vi "autoMotionProfileGenerate.vi"(11 "InputCommand":string[](array[string])) -> (2 "Acceleration steps (ft/s^2)":dbl[](array[numeric]), 3 "Speed steps (ft/s)":dbl[](array[numeric]))   [LabVIEW 2013]
panel:
  in  "autoTimeDelay":dbl
  out "Array of Computational Values":dbl[][](array[numeric])
  out "Array 2":dbl[](array[numeric])
  out "# of F2 Terms":dbl
  out "Total # of Steps":dbl
  out "# of F1 Terms":dbl
  out "N (# of steps)":dbl
  in  "T2 (s)":dbl
  in  "T1 (s)":dbl
  in  "Distance (ft)":dbl
  in  "Vprog (ft/s)":dbl
  # "Requires array slots 8, 9, 10, 11\nto be Vprog, distance, T1, T2"
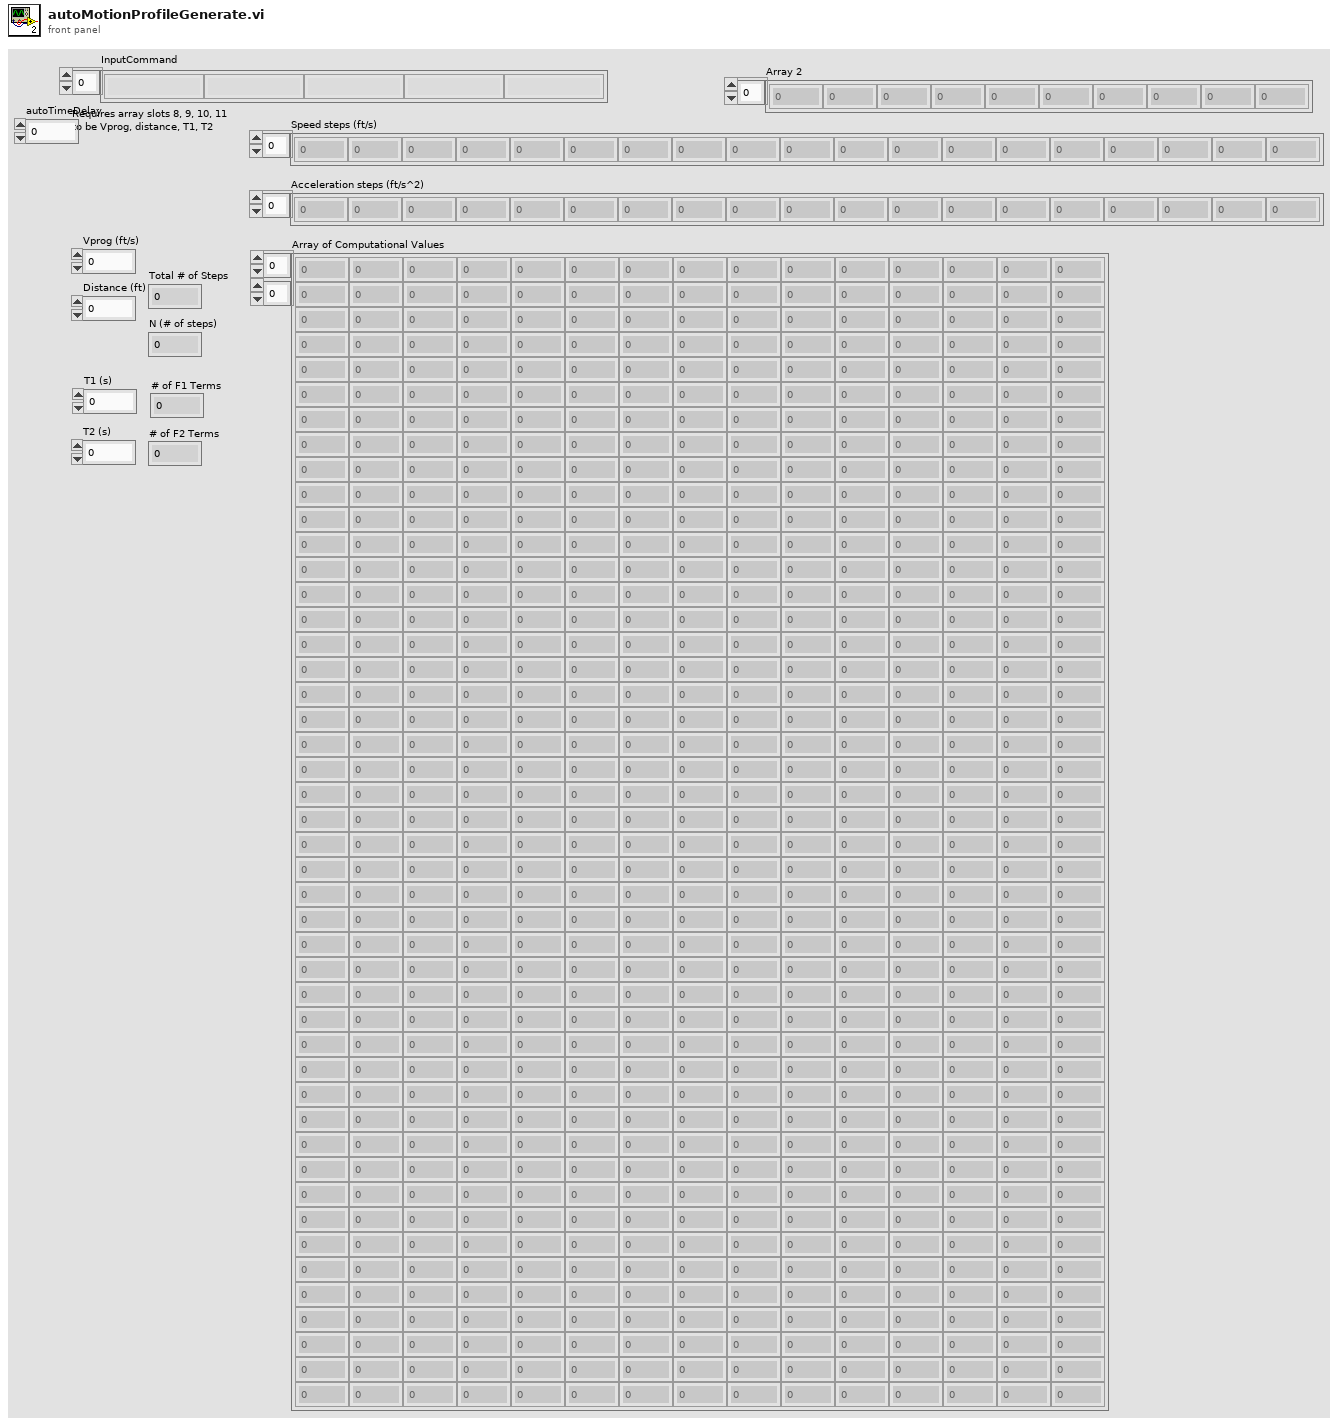
[diagram p1: front panel]
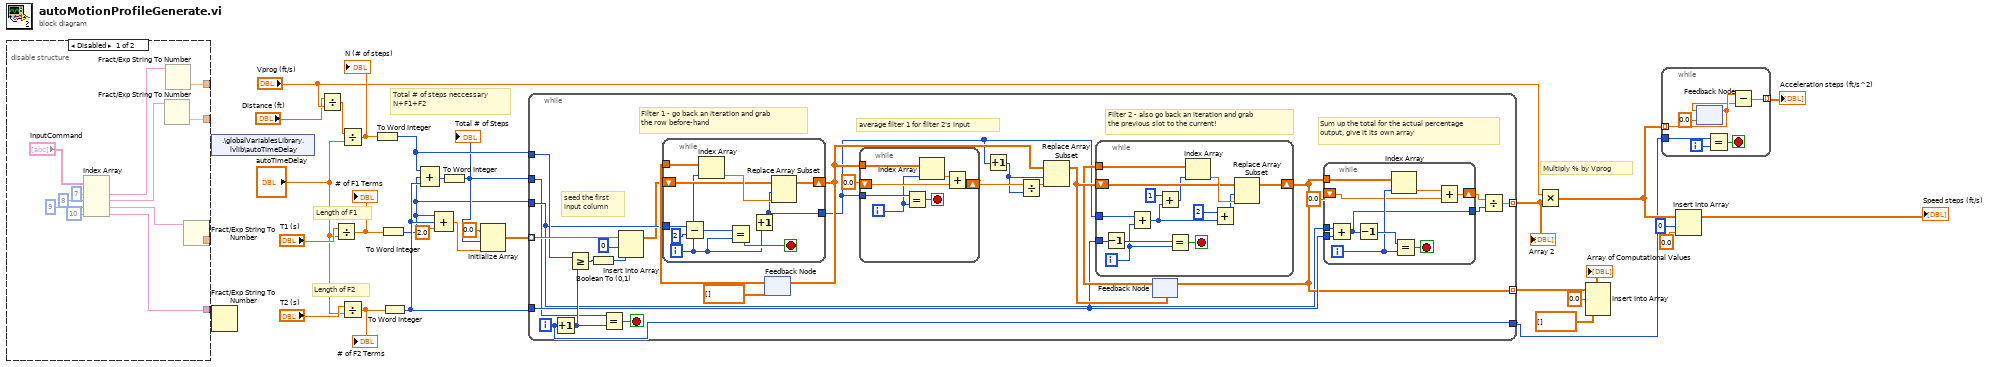
[diagram p0: block diagram]
diagram:
  # "Multiply % by Vprog"
  # "Total # of steps neccessary\nN+F1+F2"
  # "Length of F2"
  # "Length of F1"
  n1 = disable-structure shown="Disabled" {
    disable-tunnel: [w37 _] -> _
    disable-tunnel: [w36 _] -> _
    disable-tunnel: [w35 _] -> _
    disable-tunnel: [w31 _] -> w4
    frame Disabled {
      n2 = Index Array(array="InputCommand", index #1=7 ("index"), index #2=8 ("index"), index #3=9 ("index"), index #4=10 ("index")) -> (element #1=w34:string, element #2=w33:string, element #3=w32:string, element #4=w31:string)
      n3 = Fract/Exp String To Number(string=w33) -> (number=w36:dbl)  [unwired: 3 in, 1 out]
      n4 = Fract/Exp String To Number(string=w34) -> (number=w37:dbl)  [unwired: 3 in, 1 out]
      n5 = Fract/Exp String To Number(string=w32) -> (number=w35:dbl)  [unwired: 3 in, 1 out]
    }
    frame Enabled {
    }
  }
  n6 = shared-variable ".\\globalVariablesLibrary.lvlib\\autoTimeDelay"() -> ()  [unwired: 1 in, 2 out]
  n7 = Fract/Exp String To Number(string=w4) -> ()  [unwired: 3 in, 2 out]
  n8 = Divide(x="Distance (ft)", y="Vprog (ft/s)") -> (x/y=w29:dbl)
  n9 = Divide(x="T1 (s)", y="autoTimeDelay") -> (x/y=w19:dbl)
  "# of F1 Terms" <- w19
  n10 = Divide(x=w29, y="autoTimeDelay") -> (x/y=w22:dbl)
  "N (# of steps)" <- w22
  n11 = Divide(x="T2 (s)", y="autoTimeDelay") -> (x/y=w18:dbl)
  "# of F2 Terms" <- w18
  n12 = To Word Integer(number=w22) -> (16bit integer=w21:i16)
  n13 = To Word Integer(number=w19) -> (16bit integer=w12:i16)
  n14 = To Word Integer(number=w18) -> (16bit integer=w20:i16)
  n15 = Compound Arithmetic op=ADD(w21, w12, w20) -> (w24:i16)
  n16 = Compound Arithmetic op=unknown(w12, w20, 2.0 ("value")) -> (w2:dbl)
  n17 = To Word Integer(number=w24) -> (16bit integer=w17:i16)
  "Total # of Steps" <- w17
  n18 = Initialize Array(0.0, w17, w2) -> (w16:dbl[][])
  n19 = while {
    tunnel: w12 -> [w48]
    tunnel: w21 -> [w68]
    tunnel: w20 -> [w54]
    tunnel: w16 -> [w69] mode=indexing
    tunnel: [w53] -> w28 mode=indexing
    tunnel: w17 -> [w47]
    tunnel: [w50] -> w9 mode=indexing
    tunnel: [w44] -> w8
    i -> [w44]
    stop <- w43 stop-if-true
    # "Sum up the total for the actual percentage output, give it its own array"
    # "Filter 2 - also go back an iteration and grab\nthe previous slot to the current!"
    # "average filter 1 for filter 2's input"
    # "seed the first \ninput column"
    # "Filter 1 - go back an iteration and grab\nthe row before-hand"
    n20 = Increment(x=w44) -> (x+1=w67:i32)
    n21 = Greater Or Equal?(x=w68, y=w67) -> (x >= y?=w65:bool)
    n22 = Boolean To (0,1)(Boolean=w65) -> (0, 1=w66:i16)
    n23 = Equal?(x=w47, y=w67) -> (x = y?=w43:bool)
    n24 = Insert Into Array(array=w69, index=0, new element=w66) -> (w46:dbl[])
    n25 = feedback #1(dbl[] []) -> (w63:dbl[])
    n26 = while {
      shift-right: [w108] -> w62
      shift-left: w46 -> [w106]
      tunnel: w63 -> [w107]
      tunnel: w48 -> [w104]
      tunnel: [w105] -> w56
      i -> [w101]
      stop <- w110 stop-if-true
      n27 = Subtract(x=w104, y=i16 2) -> (x-y=w102:i16)
      n28 = Index Array(array=w107, index=w101) -> (element=w109:dbl)
      n29 = Equal?(x=w102, y=w101) -> (x = y?=w110:bool)
      n30 = Increment(x=w101) -> (x+1=w105:i32)
      n31 = Replace Array Subset(array=w106, new element=w109, index=w105) -> (w108:dbl[])
    }
    n32 = feedback-in #1(w62) -> ()
    n33 = while {
      tunnel: w56 -> [w95]
      tunnel: w62 -> [w96]
      shift-right: [w98] -> w61
      shift-left: 0.0 -> [w97]
      i -> [w94]
      stop <- w100 stop-if-true
      n34 = Equal?(x=w95, y=w94) -> (x = y?=w100:bool)
      n35 = Index Array(array=w96, index=w94) -> (element=w99:dbl)
      n36 = Add(x=w99, y=w97) -> (x+y=w98:dbl)
    }
    n37 = Increment(x=w56) -> (x+1=w55:i32)
    n38 = Divide(x=w61, y=w55) -> (x/y=w57:dbl)
    n39 = Replace Array Subset(array=w62, new element=w57, index=w55) -> (w59:dbl[])
    n40 = feedback #2(w59) -> (w58:dbl[])
    n41 = while {
      shift-right: [w92] -> w53
      shift-left: w59 -> [w90]
      tunnel: w58 -> [w91]
      tunnel: w56 -> [w83]
      tunnel: w54 -> [w81]
      i -> [w82]
      stop <- w85 stop-if-true
      n42 = Decrement(x=w81) -> (x-1=w84:i16)
      n43 = Add(x=w83, y=w82) -> (x+y=w80:i32)
      n44 = Add(x=i16 1, y=w80) -> (x+y=w88:i32)
      n45 = Equal?(x=w84, y=w82) -> (x = y?=w85:bool)
      n46 = Index Array(array=w91, index=w88) -> (element=w93:dbl)
      n47 = Add(x=i16 2, y=w80) -> (x+y=w86:i32)
      n48 = Replace Array Subset(array=w90, new element=w93, index=w86) -> (w92:dbl[])
    }
    n49 = feedback-in #2(w53) -> ()
    n50 = while {
      tunnel: w54 -> [w77]
      tunnel: w48 -> [w76]
      tunnel: w53 -> [w75]
      shift-right: [w72] -> w51
      shift-left: 0.0 -> [w71]
      tunnel: [w70] -> w52
      i -> [w74]
      stop <- w79 stop-if-true
      n51 = Add(x=w76, y=w77) -> (x+y=w70:i16)
      n52 = Decrement(x=w70) -> (x-1=w78:i16)
      n53 = Index Array(array=w75, index=w74) -> (element=w73:dbl)
      n54 = Equal?(x=w78, y=w74) -> (x = y?=w79:bool)
      n55 = Add(x=w73, y=w71) -> (x+y=w72:dbl)
    }
    n56 = Divide(x=w51, y=w52) -> (x/y=w50:dbl)
  }
  "Array 2" <- w9
  n57 = Multiply(x="Vprog (ft/s)", y=w9) -> (x*y=w11:dbl[])
  n58 = Insert Into Array(array=w28, index (row)=0.0, new element=dbl[] []) -> (→"Array of Computational Values":dbl[][])  [unwired: 1 in]
  n59 = while {
    tunnel: w8 -> [w117]
    tunnel: w11 -> [w114] mode=indexing
    tunnel: [w111] -> w10 mode=indexing
    i -> [w116]
    stop <- w115 stop-if-true
    n60 = feedback-in #3(w114) -> ()
    n61 = feedback #3(0.0) -> (w113:dbl)
    n62 = Equal?(x=w117, y=w116) -> (x = y?=w115:bool)
    n63 = Subtract(x=w114, y=w113) -> (x-y=w111:dbl)
  }
  "Acceleration steps (ft/s^2)" <- w10
  n64 = Insert Into Array(array=w11, index=0, new element=0.0 ("new element/subarray")) -> (→"Speed steps (ft/s)":dbl[])
